vi "Reset.vi"(8 "error in (no error)":errorcluster, 11 "NHRDCPower in":refnum<class "NHRDCPower.lvclass">) -> (0 "error out":errorcluster, 3 "NHRDCPower out":refnum<class "NHRDCPower.lvclass">)   [LabVIEW 2018, in "AcPwrPlugins.lvlib" / "NHRDCPower.lvclass"]
doc: "This VI resets the instrument(s) into a know state."
uses:
  NHRDCPower.lvclass
  <instrlib>/NHRDCPowerModule/NHRDCPowerModule/NHRDCPowerModule.lvlib
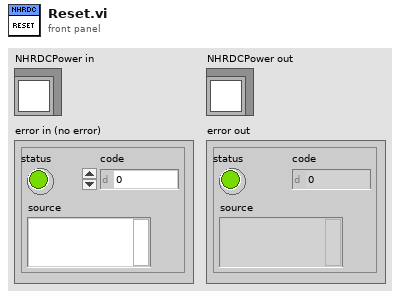
[diagram p1: front panel]
types:
  T1 = typedef "AcPwrPlugins.lvlib/NHRDCPower.lvclass/Device(s)Settings.ctl" = cluster{"MeasName":string, "Modules":T2}
  T2 = typedef "AcPwrPlugins.lvlib/NHRDCPower.lvclass/Modules.ctl" = cluster{"Handle":string, "Name":string, "id query (Yes)":bool, "reset device (Yes)":bool, "Connected":bool, "Initial Battery Detect Voltage (0)":dbl, "SafetySettings":cluster{"SetWatchDog?":bool, "Voltage (V)":dbl, "Current (A)":dbl, "Power (W)":dbl, "Voltage Delay (s)":dbl, "Current Delay (s)":dbl, "Power Delay (s)":dbl}, "Options String":string, "Aperture Time (s)":dbl, "operating state (Off)":i32, "OutputSettings":cluster{"Voltage (V)":dbl, "Current (A)":dbl, "Resistance (Ohms)":dbl, "Power (W)":dbl, "Enable Voltage":bool, "Enable Current":bool, "Enable Resistance":bool, "Enable Power":bool, "Macro After Step Delay  (s)":dbl, "Wait Value (V, A, W)":dbl, "Enable Wait":bool, "Wait on Value":i32}[], "SlewRate":cluster{"Set Voltage Rate V/S":dbl, "Set Current Rate A/S":dbl, "Set Resistance Rate R/S":dbl, "Set Power Rate W/S":dbl}, "Macro":cluster{"Save Macro?":bool, "Load Macro From File?":bool, "Run Macro Continuously?":bool, "Use Macros?":bool, "Load Macro File Path":string, "Save Macro File Path":string}, "Regulation Gain (1=100%)":dbl, "UpdatingOntheFly":bool}[]
  T3 = typedef "AcPwrPlugins.lvlib/NHRDCPower.lvclass/Measurements.ctl" = cluster{"Handle":string, "Name":string, "Enabled":bool, "Measurement Value":sgl, "Measurement Type":enum16{"Power", "Current", "Voltage"}}[]
  T4 = cluster{"Handle":string, "Name":string, "id query (Yes)":bool, "reset device (Yes)":bool, "Connected":bool, "Initial Battery Detect Voltage (0)":dbl, "SafetySettings":cluster{"SetWatchDog?":bool, "Voltage (V)":dbl, "Current (A)":dbl, "Power (W)":dbl, "Voltage Delay (s)":dbl, "Current Delay (s)":dbl, "Power Delay (s)":dbl}, "Options String":string, "Aperture Time (s)":dbl, "operating state (Off)":i32, "OutputSettings":cluster{"Voltage (V)":dbl, "Current (A)":dbl, "Resistance (Ohms)":dbl, "Power (W)":dbl, "Enable Voltage":bool, "Enable Current":bool, "Enable Resistance":bool, "Enable Power":bool, "Macro After Step Delay  (s)":dbl, "Wait Value (V, A, W)":dbl, "Enable Wait":bool, "Wait on Value":i32}[], "SlewRate":cluster{"Set Voltage Rate V/S":dbl, "Set Current Rate A/S":dbl, "Set Resistance Rate R/S":dbl, "Set Power Rate W/S":dbl}, "Macro":cluster{"Save Macro?":bool, "Load Macro From File?":bool, "Run Macro Continuously?":bool, "Use Macros?":bool, "Load Macro File Path":string, "Save Macro File Path":string}, "Regulation Gain (1=100%)":dbl, "UpdatingOntheFly":bool}
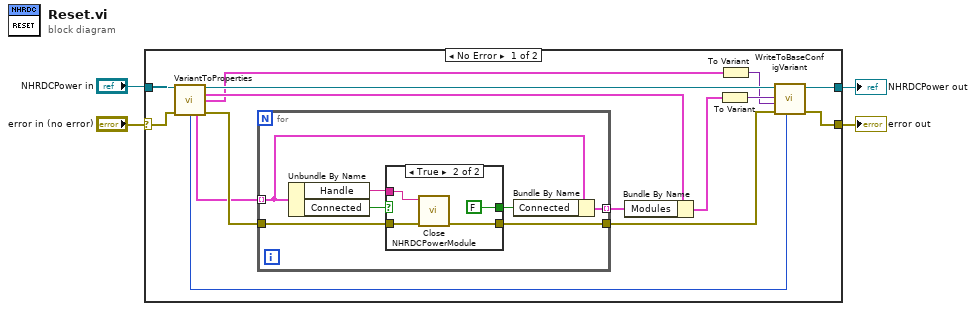
[diagram p0: block diagram]
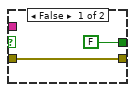
[diagram p2: hidden frame]
diagram:
  n1 = case shown="No Error" "error in (no error)" {
    selector: "error in (no error)" -> [w18 w33]
    tunnel: "NHRDCPower in" -> [w19 w34]
    tunnel: [w14 w34] -> w1
    tunnel: [w15 w33] -> w2
    frame No Error {
      n2 = call "VariantToProperties.vi"("NHRDCPower in"=w19, "error in (no error)"=w18) -> ("NHRDCPower out"=w13:refnum<class "NHRDCPower.lvclass">, "NHRDC"=w8:T1, "Meas"=w5:T3, "Measurement Refresh Time (ms)"=w7:u32, "Modules"=w11:T2, "error out"=w17:errorcluster)  [unwired: 7 in, 1 out]
      n3 = for {
        tunnel: w11 -> [w24] mode=indexing
        tunnel: w17 -> [w26]
        tunnel: [w20] -> w9 mode=indexing
        tunnel: [w25] -> w16
        n4 = Unbundle By Name(w24) -> ("Handle"=w21:string, "Connected"=w22:bool)
        n5 = case shown="True" w22 {
          tunnel: w26 -> [w28 w29]
          tunnel: [w28 w30] -> w25
          tunnel: w21 -> [_ w31]
          tunnel: [FALSE FALSE] -> w23
          frame False {
          }
          frame True {
            n6 = call <instrlib>:"Close NHRDCPowerModule.vi"("error in (no error)"=w29, "instrument handle"=w31) -> ("error out"=w30:errorcluster)  [unwired: 9 in]
          }
        }
        n7 = Bundle By Name(cluster=w24, "Connected"=w23) -> (w20:T4)
      }
      n8 = Bundle By Name(cluster=w8, "Modules"=w9) -> (w10:T1)
      n9 = To Variant(anything=w10) -> (Variant=w12:variant)
      n10 = To Variant(anything=w5) -> (Variant=w6:variant)
      n11 = call "WriteToBaseConfigVariant.vi"("Measurement Refresh Time (ms)"=w7, "error in (no error)"=w16, "Meas"=w6, "Config"=w12, "NHRDCPower in"=w13) -> ("error out"=w15:errorcluster, "NHRDCPower out"=w14:refnum<class "NHRDCPower.lvclass">)  [unwired: 5 in]
    }
    frame Error {
    }
  }
  "error out" <- w2
  "NHRDCPower out" <- w1
